vi "Role Decisor Simple.vi"(4 "id joystick":dbl, 6 "joystick in ?":bool, 11 "channel":T1) -> (3 "channel 2":T1)   [LabVIEW 2016]
uses:
  <extravilib>/ChannelInstances/Lossy Stream-t'AI Input.ctl'/)Channel.ctl
  Core/AI Input.ctl
  Core/AI Robot.ctl
  Core/AI Ball.ctl
  Core/Field Size.ctl
  Core/AI Judge.ctl
  Intel/Command Enum.ctl
  <extravilib>/ChannelInstances/Lossy Stream-t'AI Input.ctl'/Read With Abort.vi
  <extravilib>/ChannelInstances/Lossy Stream-t'AI Input.ctl'/Write With Abort.vi
  <extravilib>/ChannelInstances/Lossy Stream-t'AI Input.ctl'/Endpoint.vi
  <extravilib>/ChannelInstances/Lossy Stream-t'AI Input.ctl'/)Channel.vi
  <resource>/ChannelSupport/_ChannelSupport/WaitIfNeeded.vi
  <extravilib>/ChannelInstances/Lossy Stream-t'AI Input.ctl'.lvlib
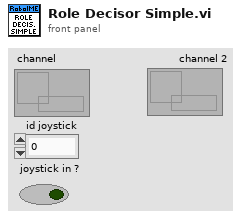
[diagram p1: front panel]
types:
  T1 = typedef "Lossy Stream-t'AI Input.ctl'.lvlib/)Channel.ctl" = refnum<queue>
  T2 = typedef "AI Input.ctl" = cluster{"our_robots":T3[], "enemy_robots":T3[], "balls":T4[], "geometry":T5, "IA Judge":T6}
  T3 = typedef "AI Robot.ctl" = cluster{"id":u32, "function":enum16{"Attacker", "Goalie", "Defender", "Joystick"}, "x":dbl, "y":dbl, "orientation":dbl, "v_tangent":dbl, "v_normal":dbl, "v_ang":dbl, "kick_x":dbl, "kick_z":dbl, "dribble":bool, "Timestamp":timestamp}
  T4 = typedef "AI Ball.ctl" = cluster{"x":dbl, "y":dbl, "timestamp":timestamp}
  T5 = typedef "Field Size.ctl" = cluster{"line_width":u32, "field_length":u32, "field_width":u32, "boundary_width":u32, "referee_width":u32, "goal_width":u32, "goal_depth":u32, "goal_wall_width":u32, "center_circle_radius":u32, "defense_radius":u32, "defense_stretch":u32, "free_kick_from_defense_dist":u32, "penalty_spot_from_field_line_dist":u32, "penalty_line_from_spot_dist":u32}
  T6 = typedef "AI Judge.ctl" = cluster{"stage":string, "command":string, "our_goalie_id":dbl, "enemy_goalie_id":dbl, "command\nenum":T7, "Time":enum16{"Azul", "Amarelo"}}
  T7 = typedef "Command Enum.ctl" = enum16{"Halt", "Stop", "Force Start", "PKA Normal Start", "Prepare Kickoff Ally", "PKE Normal Start", "Prepare Kickoff Enemy", "Prepare Penalty Ally", "Prepare Penalty Enemy", "Direct Free Enemy", "Direct Free Ally", "Indirect Free Enemy", "Indirect Free Ally", "Timeout Enemy", "Timeout Ally", "Goal Enemy", "Goal Ally", "Ball Placement Enemy", "Ball Placement Ally", "None"}
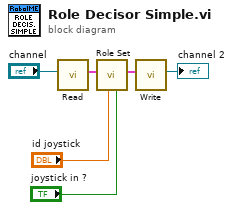
[diagram p0: block diagram]
diagram:
  n1 = call <extravilib>:"Read.vi"("channel"="channel") -> ("element"=w6:T2)  [unwired: 5 in, 5 out]
  n2 = call "Role Set.vi"("joystick in ?"="joystick in ?", "id joystick"="id joystick", "Output IA Input"=w6) -> ("Output IA"=w4:T2)  [unwired: 8 in]
  n3 = call <extravilib>:"Write.vi"("element"=w4) -> ("channel"=→"channel 2":T1)  [unwired: 8 in, 2 out]
